vi "log flow rates labjack.vi"(6 "Air Dilution Setpoint":dbl, 8 "error in":errorcluster, 9 "odor 1 setpoint":dbl, 10 "background air set point":dbl, 11 "Input Labjack Tasks":T2) -> (0 "error out":errorcluster, 2 "flow rates":T3 {"pid reading" format="%0.2f"})   [LabVIEW 2021]
uses:
  temporal odor control/LabJack Interface/LabJack AOAI Channel.ctl
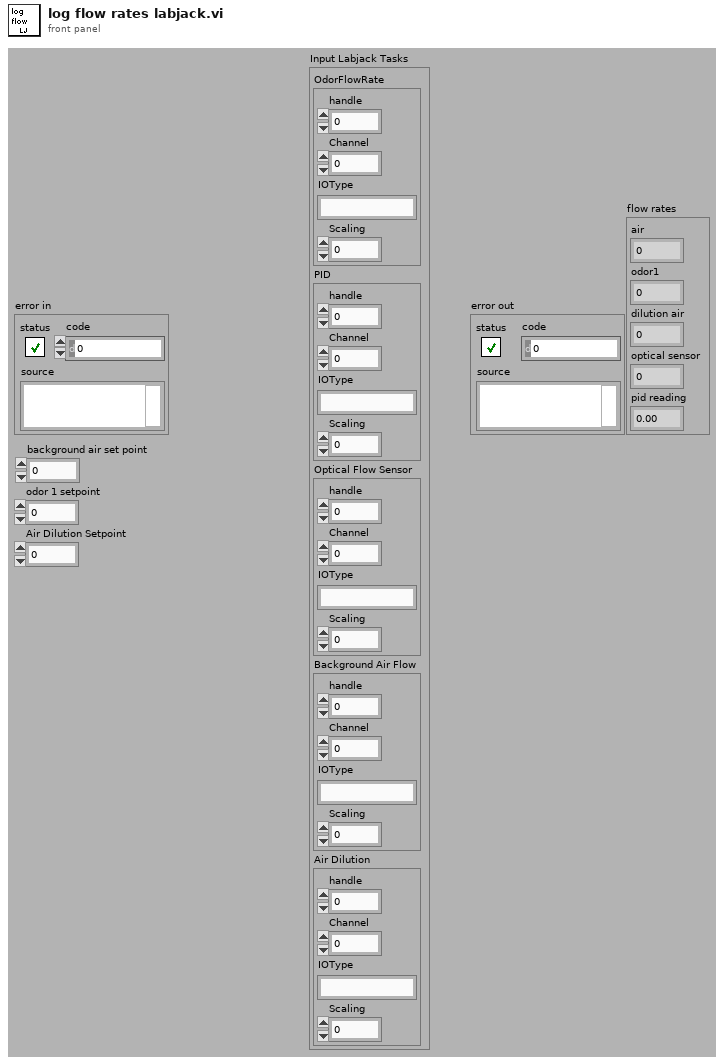
[diagram p1: front panel]
types:
  T1 = typedef "LabJack AOAI Channel.ctl" = cluster{"handle":i32, "Channel":i32, "IOType":string, "Scaling":dbl}
  T2 = cluster{"OdorFlowRate":T1, "PID":T1, "Optical Flow Sensor":T1, "Background Air Flow":T1, "Air Dilution":T1}
  T3 = cluster{"air":dbl, "odor1":dbl, "dilution air":dbl, "optical sensor":dbl, "pid reading":dbl}
  T4 = enum16{"Reset Table", "Get Values", "Add Value", "Get Table", "Get Spreadsheet", "set stack writer"}
  T5 = cluster{"[0]":dbl, "[1]":dbl, "[2]":dbl, "[3]":dbl, "[4]":dbl}
  T6 = cluster{"[3]":dbl, "[0]":dbl, "[4]":dbl, "[2]":dbl, "[1]":dbl}
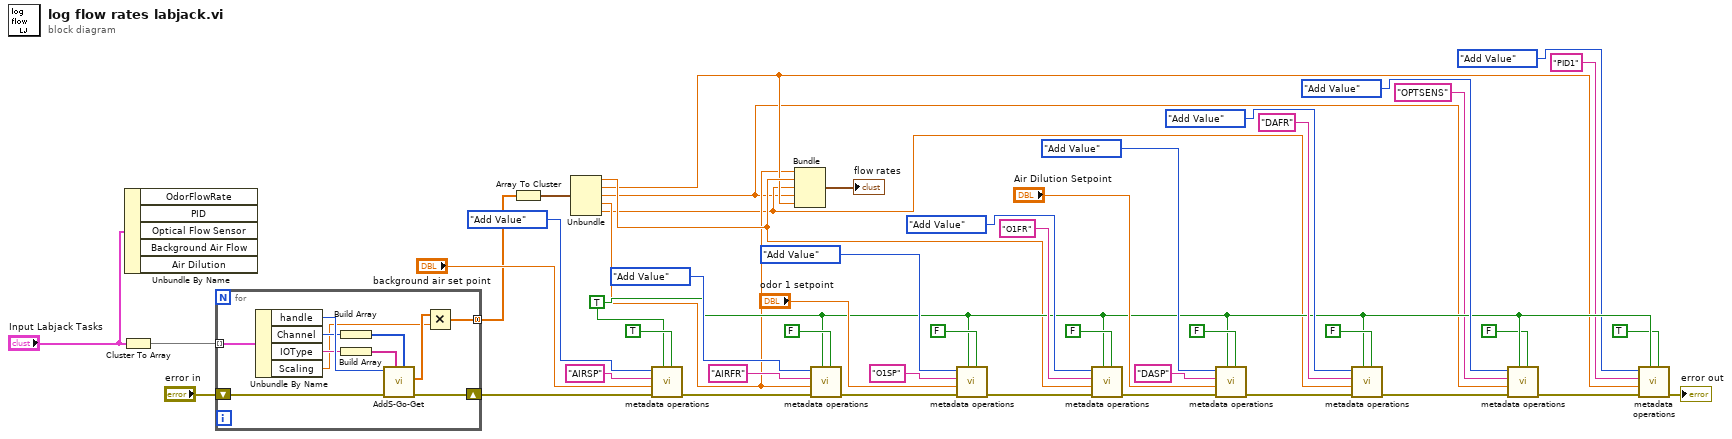
[diagram p0: block diagram]
diagram:
  w21 = TRUE ("add to stack writer")
  n1 = Cluster To Array(cluster="Input Labjack Tasks") -> (array=w16:T1[])
  n2 = Unbundle By Name("Input Labjack Tasks") -> ()  [unwired: 5 out]
  n3 = for {
    tunnel: w16 -> [w59] mode=indexing
    shift-right: [w56] -> w4
    shift-left: "error in" -> [w57]
    tunnel: [w49] -> w15 mode=concatenating
    n4 = Unbundle By Name(w59) -> ("handle"=w58:i32, "Channel"=w55:i32, "IOType"=w52:string, "Scaling"=w50:dbl)
    n5 = Build Array(w55) -> (w54:i32[])
    n6 = Build Array(w52) -> (w53:string[])
    n7 = call "AddS-Go-Get.vi"("Channels"=w54, "IOTypes"=w53, "error in"=w57, "Handle In"=w58) -> ("error out"=w56:errorcluster, "Values Read"=w51:dbl[])  [unwired: 5 in, 1 out]
    n8 = Multiply(x=w51, y=w50) -> (x*y=w49:dbl[])
  }
  n9 = Array To Cluster(array=w15) -> (cluster=w14:T5)
  n10 = Unbundle(w14) -> ("[0]"=w13:dbl, "[1]"=w9:dbl, "[2]"=w6:dbl, "[3]"=w8:dbl, "[4]"=w7:dbl)
  n11 = call "metadata operations.vi"("add time?"=TRUE, "add to stack writer"=w21, "error in (no error)"=w4, "value"="background air set point", "key"="AIRSP", "Operation"=T4."Add Value") -> ("error out"=w42:errorcluster)  [unwired: 2 in, 3 out]
  n12 = Bundle("[3]"=w8, "[0]"=w13, "[4]"=w7, "[2]"=w6, "[1]"=w9) -> (→"flow rates":T6)  [unwired: 1 in]
  n13 = call "metadata operations.vi"("add time?"=FALSE, "add to stack writer"=w21, "error in (no error)"=w42, "value"=w8, "key"="AIRFR", "Operation"=T4."Add Value") -> ("error out"=w35:errorcluster)  [unwired: 2 in, 3 out]
  n14 = call "metadata operations.vi"("add time?"=FALSE, "add to stack writer"=w21, "error in (no error)"=w35, "value"="odor 1 setpoint", "key"="O1SP", "Operation"=T4."Add Value") -> ("error out"=w36:errorcluster)  [unwired: 2 in, 3 out]
  n15 = call "metadata operations.vi"("add time?"=FALSE, "add to stack writer"=w21, "error in (no error)"=w36, "value"=w13, "key"="O1FR", "Operation"=T4."Add Value") -> ("error out"=w28:errorcluster)  [unwired: 2 in, 3 out]
  n16 = call "metadata operations.vi"("add time?"=FALSE, "add to stack writer"=w21, "error in (no error)"=w28, "value"="Air Dilution Setpoint", "key"="DASP", "Operation"=T4."Add Value") -> ("error out"=w29:errorcluster)  [unwired: 2 in, 3 out]
  n17 = call "metadata operations.vi"("add time?"=FALSE, "add to stack writer"=w21, "error in (no error)"=w29, "value"=w7, "key"="DAFR", "Operation"=T4."Add Value") -> ("error out"=w3:errorcluster)  [unwired: 2 in, 3 out]
  n18 = call "metadata operations.vi"("add time?"=FALSE, "add to stack writer"=w21, "error in (no error)"=w3, "value"=w6, "key"="OPTSENS", "Operation"=T4."Add Value") -> ("error out"=w2:errorcluster)  [unwired: 2 in, 3 out]
  n19 = call "metadata operations.vi"("add time?"=TRUE, "add to stack writer"=w21, "error in (no error)"=w2, "value"=w9, "key"="PID1", "Operation"=T4."Add Value") -> ("error out"=→"error out":errorcluster)  [unwired: 2 in, 3 out]
